vi "Operator Dialog for Key Press Platinum.vi"() -> ()   [LabVIEW 2024, in "VehicleModelPlatinum.lvclass"]
uses:
  VehicleModelPlatinum.lvclass
  VehicleModelPlatinum.lvclass/VehicleModelPlatinum.ctl
panel:
  in  "Boolean":bool
  # "Press KeyFob Platinum"
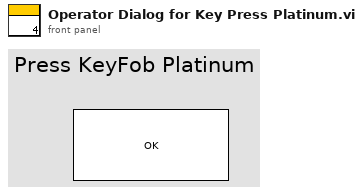
[diagram p1: front panel]
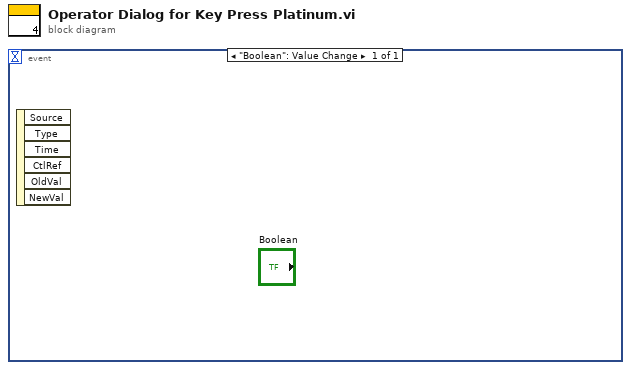
[diagram p0: block diagram]
diagram:
  n1 = event shown="[0] \"Boolean\": Value Change" {
    selector: _ -> [_]
    dyn-events: _ -> [_]
    timeout: _ -> [_]
    event "Boolean": Value Change {
      n2 = event-data() -> ()  [unwired: 1 in, 6 out]
    }
  }
